vi "test Multi FPGA Synchronization.vi"(8 "error in (no error)":errorcluster, 11 "TestCase in":refnum<class "Engine Simulation Multi FPGA System Tests.lvclass">) -> (0 "error out":errorcluster, 3 "TestCase out":refnum<class "Engine Simulation Multi FPGA System Tests.lvclass">)   [LabVIEW 2015, in "Engine Simulation Multi FPGA System Tests.lvclass"]
uses:
  Engine Simulation Multi FPGA System Tests.lvclass
  <vilib>/NI Veristand/Execution/Workspace/NI VeriStand - Set Single Channel Value.vi
  <vilib>/NI Veristand/Execution/Workspace/NI VeriStand - Get Multiple Channel Values.vi
  <vilib>/addons/_JKI Toolkits/VI Tester/TestCase.llb/TestCase.lvclass
  <vilib>/NI Veristand/Execution/Workspace/NI_VS Workspace ExecutionAPI.lvlib
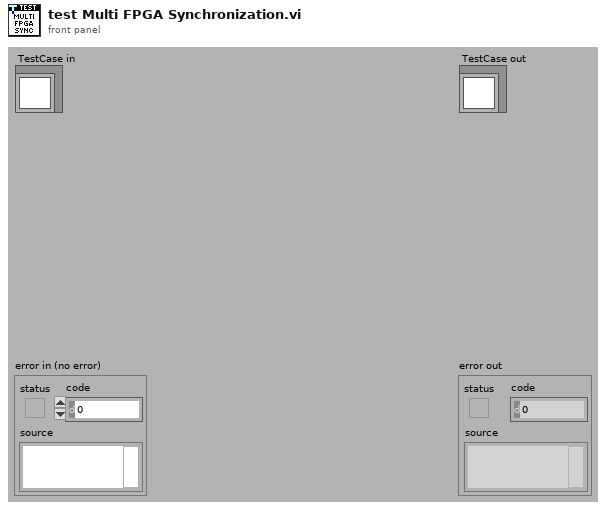
[diagram p1: front panel]
types:
  T1 = typedef "NI_VS Workspace ExecutionAPI.lvlib/WorkspaceAPI.ctl" = refnum<k24>
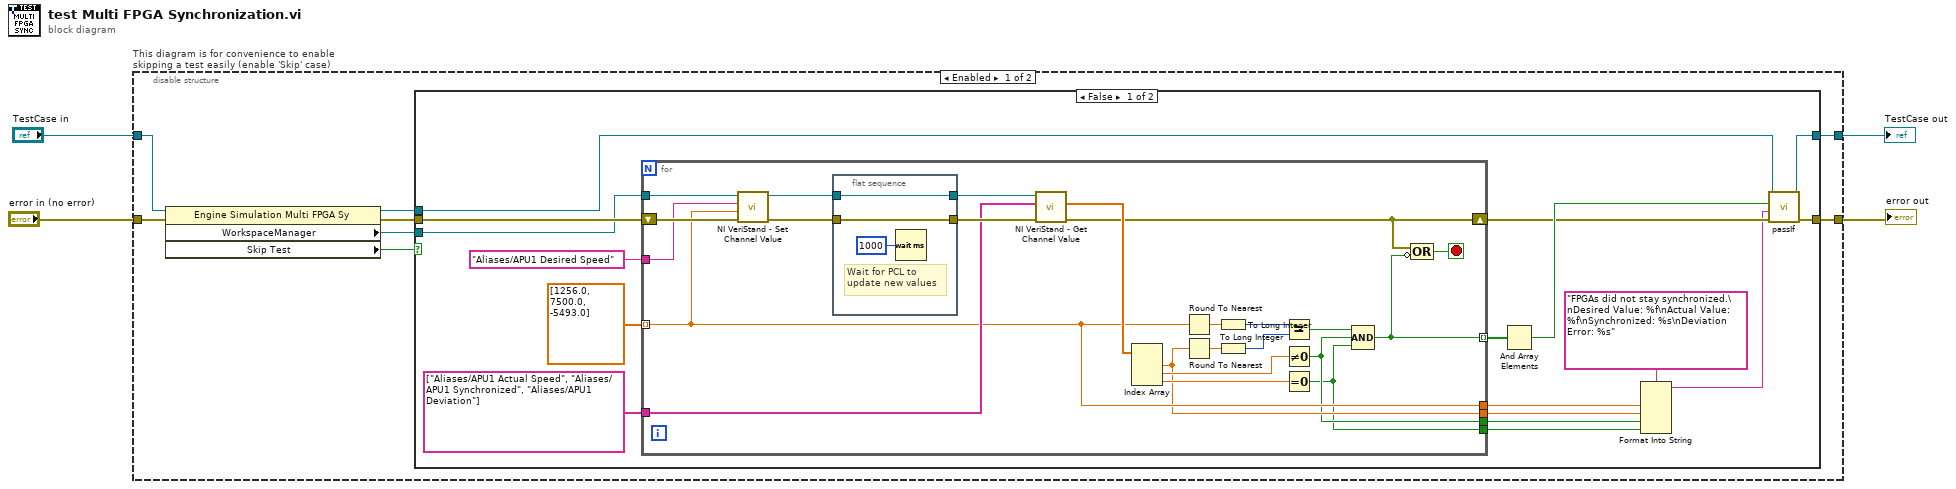
[diagram p0: block diagram]
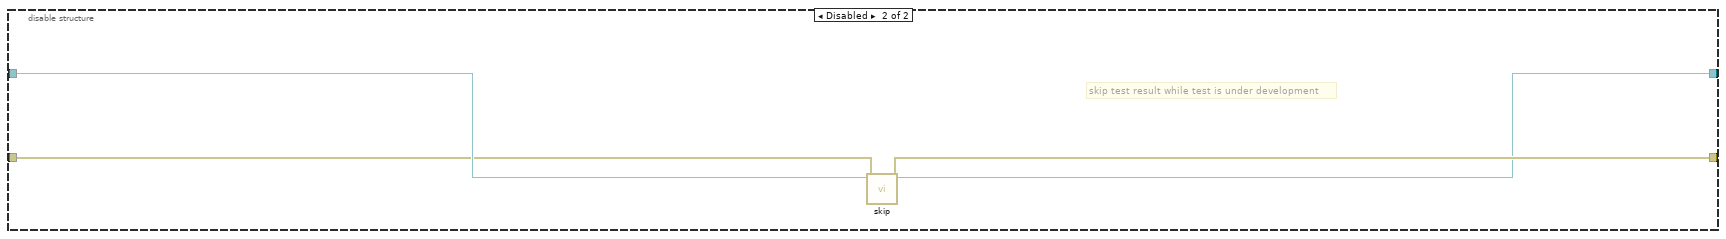
[diagram p3: hidden frame]
diagram:
  n1 = disable-structure "This diagram is for convenience to enable skipping a test easily (enable 'Skip' case)" shown="Enabled" {
    disable-tunnel: "TestCase in" -> [w12 w61]
    disable-tunnel: [w7 w59] -> w1
    disable-tunnel: [w6 w60] -> w3
    disable-tunnel: "error in (no error)" -> [w11 w58]
    frame Enabled {
      n2 = property class="Engine Simulation Multi FPGA Sy"(reference=w12, error in=w11) -> (reference out=w8:refnum<class "Engine Simulation Multi FPGA System Tests.lvclass">, error out=w10:errorcluster, "WorkspaceManager"=w9:T1, "Skip Test"=w5:bool)
      n3 = case shown="False" w5 {
        tunnel: w10 -> [w29 w57]
        tunnel: w9 -> [w28 _]
        tunnel: w8 -> [w22 w56]
        tunnel: [w21 w56] -> w7
        tunnel: [w19 w57] -> w6
        frame False {
          n4 = for {
            tunnel: "Aliases/APU1 Desired Speed" -> [w50]
            shift-right: [w35] -> w20
            shift-left: w29 -> [w52]
            tunnel: dbl[] [1256.0, 7500.0, -5493.0] -> [w33] mode=indexing
            tunnel: string[] ["Aliases/APU1 Actual Speed", "Aliases/APU1 Synchronized", "Aliases/APU1 Deviation"] -> [w38]
            tunnel: w28 -> [w51]
            tunnel: [w36] -> w24 mode=indexing
            tunnel: [w33] -> w17
            tunnel: [w32] -> w16
            tunnel: [w31] -> w15
            tunnel: [w30] -> w14
            stop <- w34 stop-if-true
            n5 = call-poly <vilib>:"NI VeriStand - Set Channel Value.vi"("error in (no error)"=w52, "Value"=w33, "Channel"=w50, "WorkspaceManager in"=w51) -> ("error out"=w40:errorcluster, "WorkspaceManager out"=w39:T1)  [unwired: 6 in]
            n6 = flat-sequence {
              tunnel: w39 -> [w54]
              tunnel: w40 -> [w55]
              tunnel: [w55] -> w43
              tunnel: [w54] -> w42
              frame #0 {
                # "Wait for PCL to\nupdate new values"
                n7 = Wait (ms)(milliseconds to wait=u32 1000) -> ()  [unwired: 1 out]
              }
            }
            n8 = call-poly <vilib>:"NI VeriStand - Get Channel Value.vi"("error in (no error)"=w43, "Channels"=w38, "WorkspaceManager in"=w42) -> ("error out"=w35:errorcluster, "Values"=w49:dbl[])  [unwired: 6 in, 1 out]
            n9 = Index Array(array=w49) -> (element #1=w32:dbl, element #2=w48:dbl, element #3=w47:dbl)  [unwired: 3 in]
            n10 = Round To Nearest(number=w33) -> (nearest integer value=w45:dbl)
            n11 = Round To Nearest(number=w32) -> (nearest integer value=w44:dbl)
            n12 = To Long Integer(number=w45) -> (32bit integer=w41:i32)
            n13 = To Long Integer(number=w44) -> (32bit integer=w37:i32)
            n14 = Equal?(x=w41, y=w37) -> (x = y?=w46:bool)
            n15 = Not Equal To 0?(x=w48) -> (x != 0?=w31:bool)
            n16 = Equal To 0?(x=w47) -> (x = 0?=w30:bool)
            n17 = Compound Arithmetic op=AND(w46, w31, w30) -> (w36:bool)
            n18 = Compound Arithmetic op=OR(w35, invert w36) -> (w34:bool)
          }
          n19 = And Array Elements(Boolean array=w24) -> (logical AND=w23:bool)
          n20 = Format Into String(format string="FPGAs did not stay synchronized.\nDesired Value: %f\nActual Value: %f\nSynchronized: %s\nDeviation Error: %s", w17, w16, w15, w14) -> (resulting string=w13:string)  [unwired: 2 in, 1 out]
          n21 = call-dynamic "passIf.vi"("error in (no error)"=w20, "message (\"\")"=w13, "pass"=w23, "TestCase in"=w22) -> ("error out"=w19:errorcluster, "TestCase out"=w21:refnum<class "Engine Simulation Multi FPGA System Tests.lvclass">)  [unwired: 6 in]
        }
        frame True {
        }
      }
    }
    frame Disabled {
      # "skip test result while test is under development"
      n22 = call <vilib>:"skip.vi"("error in (no error)"=w58, "TestCase in"=w61) -> ("error out"=w60:errorcluster, "TestCase out"=w59:refnum<class "Engine Simulation Multi FPGA System Tests.lvclass">)  [unwired: 8 in]
    }
  }
  "error out" <- w3
  "TestCase out" <- w1
